vi "prova espotrazione excel.vi"() -> ()   [LabVIEW 2019]
uses:
  <vilib>/Utility/NIReport.llb/NI_report.lvclass
panel:
  in  "template (empty)":path
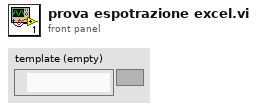
[diagram p1: front panel]
types:
  T1 = enum16{"maximized", "minimized", "normal", "no change"}
  T2 = enum16{"Standard Report", "HTML", "Word", "Excel"}
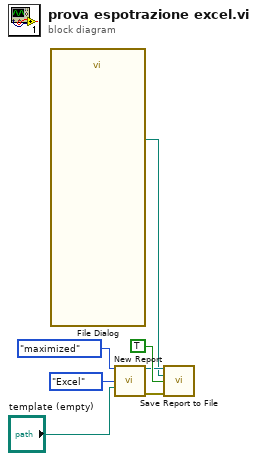
[diagram p0: block diagram]
diagram:
  n1 = call "File Dialog"() -> ("selected path"=w1:path)  [unwired: 7 in, 8 out]
  n2 = call <vilib>:"New Report.vi"("window state (normal)"=T1."maximized", "report type"=T2."Excel", "template (empty)"="template (empty)") -> ("report out"=w3:refnum<class "NI_report.lvclass">, "error out"=w2:errorcluster)  [unwired: 11 in]
  n3 = call-dynamic "Save Report to File.vi"("report in"=w3, "report file path"=w1, "prompt to replace? (F)"=TRUE, "error in (no error)"=w2) -> ()  [unwired: 10 in, 2 out]
